vi "Set Range.vi"(6 "Control Ref Queue":T1, 8 "error in (no error)":errorcluster, 10 "Multiplot Representation In":T2, 11 "2D Compass.lvclass in":refnum<class "2D Compass.lvclass">) -> (0 "error out":errorcluster, 2 "Multiplot Representation Out":T2, 3 "2D Compass.lvclass out":refnum<class "2D Compass.lvclass">)   [LabVIEW 2020, in "2D Compass.lvclass"]
uses:
  <vilib>/Math Plots/2D Math Plots/2D Compass/2D Compass/2D Compass.lvclass
  e:/builds/penguin/labview/branches/2020/dev/dist/vi.lib/Math Plots/2D Math Plots/2D Plot/2D Plot/2D Plot.lvclass
  <vilib>/Math Plots/2D Math Plots/2D Plot/2D Plot/Typedef/Multiplot Representation.ctl
  <vilib>/Math Plots/2D Math Plots/2D Plot/2D Plot/Typedef/Plot Representation.ctl
  <vilib>/Math Plots/2D Math Plots/2D Plot/2D Plot/Typedef/Range Cluster.ctl
  <vilib>/Math Plots/2D Math Plots/2D Plot/Action String/2DMathPlot Ctrl Act Queue.ctl
  <vilib>/Math Plots/2D Math Plots/2D Plot/Action String/2DMathPlot Ctrl Act Cluster.ctl
  <vilib>/Math Plots/2D Math Plots/2D Plot/Action String/2DMathPlot State Class.ctl
  <vilib>/Math Plots/2D Math Plots/2D Plot/2D Plot/2D Plot.lvclass
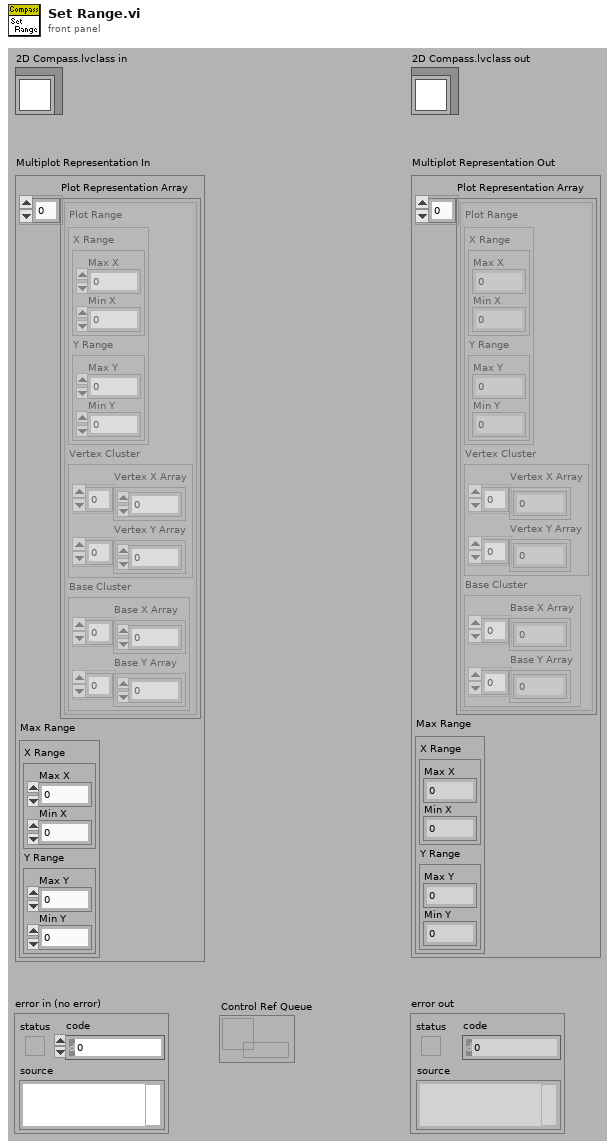
[diagram p1: front panel]
types:
  T1 = typedef "2DMathPlot Ctrl Act Queue.ctl" = refnum<queue>
  T2 = typedef "2D Plot.lvclass/Multiplot Representation.ctl" = cluster{"Plot Representation Array":T3[], "Max Range":T4}
  T3 = typedef "2D Plot.lvclass/Plot Representation.ctl" = cluster{"Plot Range":T4, "Vertex Cluster":cluster{"Vertex X Array":dbl[], "Vertex Y Array":dbl[]}, "Base Cluster":cluster{"Base X Array":dbl[], "Base Y Array":dbl[]}}
  T4 = typedef "2D Plot.lvclass/Range Cluster.ctl" = cluster{"X Range":cluster{"Max X":dbl, "Min X":dbl}, "Y Range":cluster{"Max Y":dbl, "Min Y":dbl}}
  T5 = typedef "2D Plot.lvclass/Property Cluster.ctl" = cluster{"Graph General":T6, "Format Property":string[], "Scale Array":T7, "Cursor Property":T10, "Annotation List":T12, "Active Cursor":i32, "Active Plot":i32}
  T6 = typedef "2D Plot.lvclass/Graph General Property.ctl" = cluster{"Palette Visible":cluster{"Graph Legend":bool, "Plot Legend":bool, "Auto size":bool, "Number of Plots":u32, "X Scrollbar":bool, "Scale Legend":bool, "Cursor Legend":bool}, "Plot Area Color":cluster{"FG Color":u32, "BG Color":u32}, "Bounds Size":cluster{"Width":u32, "Height":u32}, "Plot Area Bounds":cluster{"Left":i16, "Top":i16, "Right":i16, "Bottom":i16}}
  T7 = typedef "2D Plot.lvclass/Scale Array.ctl" = T8[]
  T8 = typedef "2D Plot.lvclass/Scale Cluster.ctl" = cluster{"General":cluster{"Editable":bool, "Flipped":bool, "Mapping Mode":u8, "Visible":bool, "Style":u8, "Scale Fit":u8}, "Offset and Multiplier":T9, "Range":cluster{"Minimum":dbl, "Maximum":dbl, "Increment":dbl, "Minor Increment":dbl, "Start":dbl}, "Tick Color":cluster{"Major Color":u32, "Minor Color":u32}, "Gird Color":cluster{"Major Color":u32, "Minor Color":u32}, "Marker":cluster{"Visible":bool, "FG Color":u32, "BG Color":u32, "Font Name":string, "Font Size":u32, "Font Bold":bool, "Font Italic":bool, "Font Strikeout":bool, "Font Underline":bool}, "Name Label":cluster{"Visible":bool, "FG Color":u32, "BG Color":u32, "Font Name":string, "Font Size":u32, "Font Bold":bool, "Font Italic":bool, "Font Strikeout":bool, "Font Underline":bool, "Justification":enum16{"Left", "Center", "Right"}, "Text":string}}
  T9 = typedef "LVOffsetAndMultiplierTypeDef.ctl" = cluster{"Offset":dbl, "Multiplier":dbl}
  T10 = typedef "2D Plot.lvclass/Cursor Property.ctl" = cluster{"Cursor List":T11, "Cursor List Addtional":cluster{"Cursor Selection Color":u32, "Line Style":u8, "Line Width":u8, "Visible":bool}[]}
  T11 = typedef "LVCursorListTypeDef.ctl" = cluster{"Name":string, "Color":u32, "Style":u8, "Point Style":u8, "Name Visible":bool, "Allow Drag":bool, "Cursor Mode":u32, "Plot":i32, "Index":i32, "Position":cluster{"X":dbl, "Y":dbl}, "X Scale":u32, "Y Scale":u32, "Watch Plots":i32[], "Watch All Plots":bool, "Plot Area":i32, "Label Offset":cluster{"X":dbl, "Y":dbl}}[]
  T12 = typedef "LVAnnotationListTypeDef.ctl" = cluster{"Name":string, "Color":u32, "Style":u8, "Point Style":u8, "Name Visible":bool, "Allow Drag":bool, "Annotation Mode":u32, "Plot":i32, "Index":i32, "Position":cluster{"X":dbl, "Y":dbl}, "X Scale":u32, "Y Scale":u32, "Show Arrow":bool, "Lock Name":bool, "Plot Area":i32, "Label Offset":cluster{"X":dbl, "Y":dbl}}[]
  T13 = typedef "2DMathPlot Ctrl Act Cluster.ctl" = cluster{"Plot Area Ref":refnum<vi>, "Z Axis Ref":refnum<vi>, "Legend Ref":refnum<vi>, "XControl Ref":refnum<vi>, "Facade Ref":refnum<vi>, "Display State Change Class":T14}
  T14 = typedef "2DMathPlot State Class.ctl" = enum16{"Update All (Undo)", "Update General", "Update Appearance", "Update Format", "Update Scale", "Update Marker", "Update Cursor", "None"}
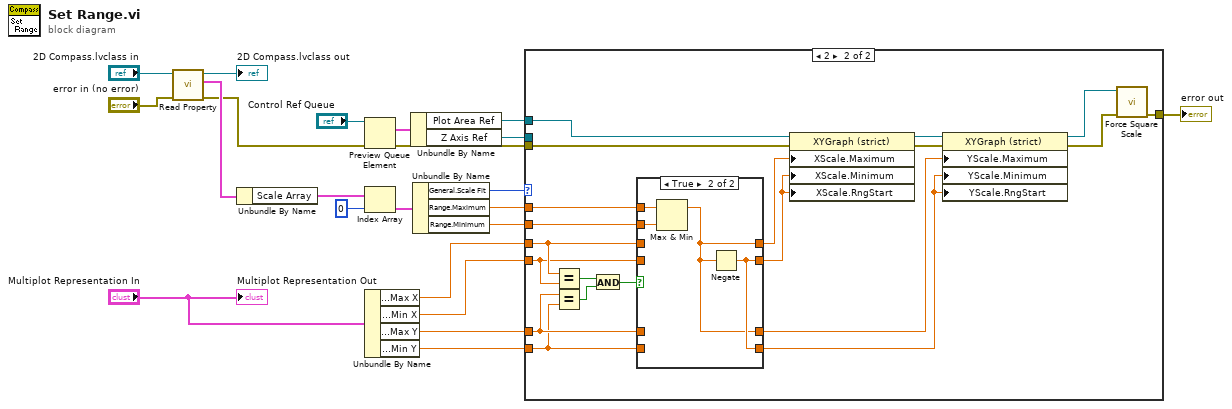
[diagram p0: block diagram]
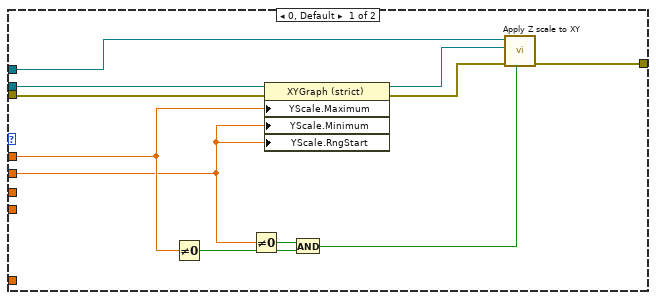
[diagram p2: hidden frame]
diagram:
  n1 = call <vilib>:"Read Property.vi"("error in (no error)"="error in (no error)", "2D Plot.lvclass in"="2D Compass.lvclass in") -> ("error out"=w15:errorcluster, "XY Graph Property Cluster"=w16:T5, "2D Plot.lvclass out"=→"2D Compass.lvclass out":refnum<class "2D Compass.lvclass">)  [unwired: 7 out]
  n2 = Unbundle By Name(w16) -> ("Scale Array"=w13:T7)
  n3 = Preview Queue Element(queue="Control Ref Queue", error in (no error)=w15) -> (element=w17:T13, error out=w8:errorcluster)  [unwired: 3 out]
  n4 = Index Array(array=w13, index=0) -> (element=w18:T8)
  n5 = Unbundle By Name("Multiplot Representation In") -> ("Max Range.X Range.Max X"=w12:dbl, "Max Range.X Range.Min X"=w11:dbl, "Max Range.Y Range.Max Y"=w9:dbl, "Max Range.Y Range.Min Y"=w10:dbl)
  n6 = Unbundle By Name(w17) -> ("Plot Area Ref"=w3:refnum<vi>, "Z Axis Ref"=w2:refnum<vi>)
  n7 = Unbundle By Name(w18) -> ("General.Scale Fit"=w6:u8, "Range.Maximum"=w5:dbl, "Range.Minimum"=w1:dbl)
  n8 = case shown="2" w6 {
    tunnel: [w32 w53] -> w22
    tunnel: w12 -> [_ w43]
    tunnel: w11 -> [_ w41]
    tunnel: w10 -> [_ w37]
    tunnel: w9 -> [_ w39]
    tunnel: w3 -> [w29 w50]
    tunnel: w8 -> [w28 w49]
    tunnel: w5 -> [w25 w35]
    tunnel: w2 -> [w31 _]
    tunnel: w1 -> [w24 w34]
    frame 0, Default {
      n9 = Not Equal To 0?(x=w25) -> (x != 0?=w27:bool)
      n10 = Not Equal To 0?(x=w24) -> (x != 0?=w26:bool)
      n11 = property class="XYGraph (strict)"(reference=w31, error in=w28, "YScale.Maximum"=w25, "YScale.Minimum"=w24, "YScale.RngStart"=w24) -> (reference out=w30:refnum<vi>, error out=w33:errorcluster)
      n12 = And(x=w26, y=w27) -> (x .and. y?=w23:bool)
      n13 = call <vilib>:"Apply Z scale to XY.vi"("Enlarge Z scale?"=w23, "error in (no error)"=w33, "Z Axis Ref"=w30, "Plot Area Ref"=w29) -> ("error out"=w32:errorcluster)  [unwired: 7 in]
    }
    frame 2 {
      n14 = Equal?(x=w43, y=w41) -> (x = y?=w45:bool)
      n15 = Equal?(x=w39, y=w37) -> (x = y?=w46:bool)
      n16 = And(x=w45, y=w46) -> (x .and. y?=w36:bool)
      n17 = case shown="True" w36 {
        tunnel: [w57 w58] -> w44
        tunnel: w43 -> [w57 _]
        tunnel: [w56 w59] -> w42
        tunnel: w41 -> [w56 _]
        tunnel: [w55 w58] -> w40
        tunnel: w39 -> [w55 _]
        tunnel: [w54 w59] -> w38
        tunnel: w37 -> [w54 _]
        tunnel: w35 -> [_ w61]
        tunnel: w34 -> [_ w60]
        frame False {
        }
        frame True {
          n18 = Max & Min(x=w61, y=w60) -> (max(x,y)=w58:dbl)  [unwired: 1 out]
          n19 = Negate(x=w58) -> (-x=w59:dbl)
        }
      }
      n20 = property class="XYGraph (strict)"(reference=w50, error in=w49, "XScale.Maximum"=w44, "XScale.Minimum"=w42, "XScale.RngStart"=w42) -> (reference out=w52:refnum<vi>, error out=w51:errorcluster)
      n21 = property class="XYGraph (strict)"(reference=w52, error in=w51, "YScale.Maximum"=w40, "YScale.Minimum"=w38, "YScale.RngStart"=w38) -> (reference out=w47:refnum<vi>, error out=w48:errorcluster)
      n22 = call <vilib>:"Force Square Scale.vi"("error in (no error)"=w48, "Plot Area Ref"=w47) -> ("error out"=w53:errorcluster)  [unwired: 1 in, 8 out]
    }
  }
  "error out" <- w22
  "Multiplot Representation Out" <- "Multiplot Representation In"
